vi "Handle Last Ack Core.vi"(4 "error in (no error)":errorcluster, 6 "Last Ack":refnum<class "Last Ack.lvclass">, 7 "Assert Startup UI in":refnum<class "Assert Startup UI.lvclass">) -> (0 "error out":errorcluster, 3 "Assert Startup UI out":refnum<class "Assert Startup UI.lvclass">)   [LabVIEW 2016, in "Assert API Components.lvlib" / "Assert Startup UI.lvlib" / "Assert Startup UI.lvclass"]
doc: "(<B>Filename</B>: Actor Framework.lvlib:Actor.lvclass:Handle Last Ack Core.vi)\n\nDefines how the caller actor responds to the Last Ack message from a nested actor. The Last Ack message is the final message a nested actor sends to its caller before it shuts down. The message contains information about the final state of the nested actor.\n\nBy default, this method does nothing except return any error the nested actor sent. A descendant class may override this method to define behavior."
uses:
  Assert Startup UI.lvclass
  <vilib>/ActorFramework/LastAck/Last Ack.lvclass
  Assert Display/Assert Display/Assert Display.lvclass
  Assert API Components/Display Type.ctl
  <vilib>/ActorFramework/LastAck/Last Ack.lvclass/Last Ack.ctl
  Assert Display/Assert Display/Assert Display.lvclass/Assert Display.ctl
  Assert Startup UI.lvclass/Assert Startup UI.ctl
  Base UI Actor/Base UI Actor/Base UI Actor.lvclass
  Assert API Components/Assert API Components.lvlib
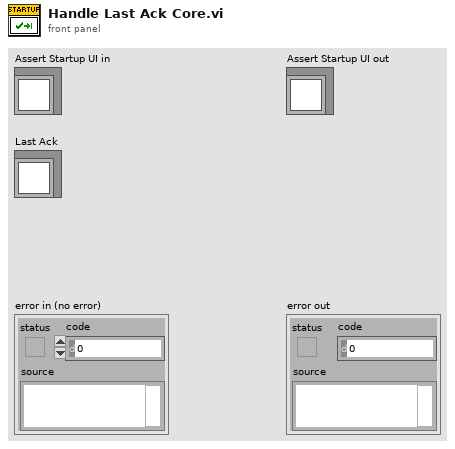
[diagram p1: front panel]
types:
  T1 = typedef "Assert API Components.lvlib/Display Type.ctl" = enum16{"Local", "Network"}
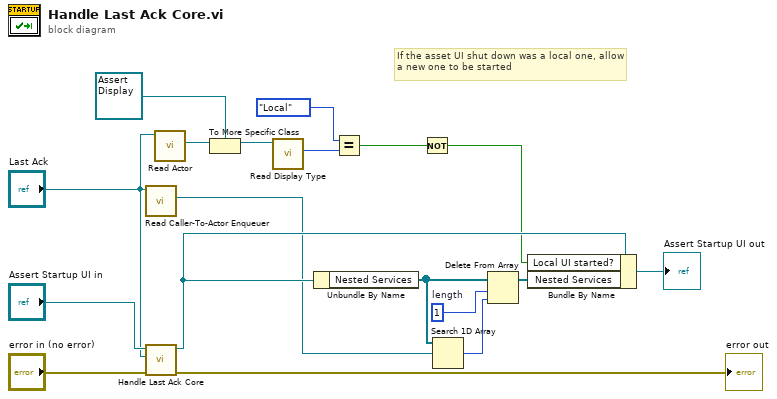
[diagram p0: block diagram]
diagram:
  w12 = 1  # length
  # "If the asset UI shut down was a local one, allow a new one to be started"
  n1 = call <vilib>:"Read Caller-To-Actor Enqueuer.vi"("Last Ack"="Last Ack") -> ("Caller-to-Actor Enqueuer"=w14:refnum<class "Message Enqueuer.lvclass">)  [unwired: 10 in]
  n2 = call-parent "Handle Last Ack Core.vi"("error in (no error)"="error in (no error)", "Last Ack"="Last Ack", "Actor in"="Assert Startup UI in") -> ("error out"=→"error out":errorcluster, "Actor out"=w15:refnum<class "Assert Startup UI.lvclass">)  [unwired: 3 in]
  n3 = call <vilib>:"Read Actor.vi"("Last Ack"="Last Ack") -> ("Actor"=w6:refnum<class "Actor.lvclass">)  [unwired: 10 in]
  n4 = To More Specific Class(target class=refnum<class "Assert Display.lvclass"> refnum ("Assert API Components.lvlib:Assert Display.lvlib:Assert Display.lvclass"), reference=w6) -> (specific class reference=w5:refnum<class "Assert Display.lvclass">)  [unwired: 1 in, 1 out]
  n5 = call "Read Display Type.vi"("Assert Display in"=w5) -> ("Display Type"=w4:T1)  [unwired: 10 in]
  n6 = Unbundle By Name(w15) -> ("Nested Services"=w13:refnum<class "Message Enqueuer.lvclass">[])
  n7 = Equal?(x=Display_Type."Local" ("Display Type"), y=w4) -> (x = y?=w2:bool)
  n8 = Not(x=w2) -> (.not. x?=w1:bool)
  n9 = Search 1D Array(1D array=w13, element=w14) -> (index of element=w11:i32)  [unwired: 1 in]
  n10 = Delete From Array(array=w13, length=w12, index=w11) -> (array with subset deleted=w9:refnum<class "Message Enqueuer.lvclass">[])  [unwired: 1 out]
  n11 = Bundle By Name(cluster=w15, "Local UI started?"=w1, "Nested Services"=w9) -> (→"Assert Startup UI out":refnum<class "Assert Startup UI.lvclass">)
